vi "Angle Correction PID.vi"(8 "I gain":dbl, 9 "D gain":dbl, 10 "P gain":dbl, 11 "Error In":dbl) -> (3 "Output":dbl)   [LabVIEW 2013, in "ProcessorHelperFunctions.lvlib"]
uses:
  ProcessorHelperFunctions.lvlib
panel:
  out "Error Input":dbl
  out "I accumulated":dbl
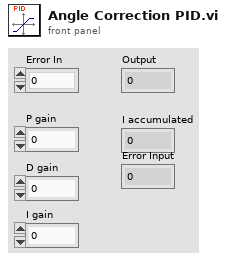
[diagram p1: front panel]
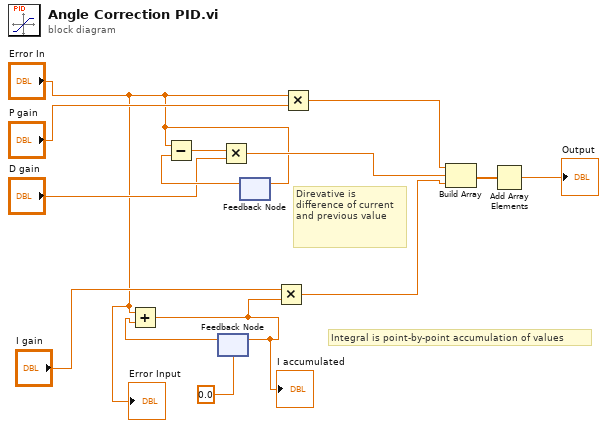
[diagram p0: block diagram]
diagram:
  # "Direvative is difference of current and previous value"
  # "Integral is point-by-point accumulation of values"
  n1 = feedback #1(0.0) -> (w6:dbl)
  n2 = Add(x="Error In", y=w6) -> (x+y=w3:dbl)
  "I accumulated" <- w3
  n3 = feedback-in #1(w3) -> ()
  n4 = feedback-in #2("Error In") -> ()
  n5 = feedback #2() -> (w10:dbl)  [unwired: 1 in]
  n6 = Subtract(x="Error In", y=w10) -> (x-y=w9:dbl)
  n7 = Multiply(x=w9, y="D gain") -> (x*y=w7:dbl)
  n8 = Multiply(x="I gain", y=w3) -> (x*y=w4:dbl)
  n9 = Multiply(x="Error In", y="P gain") -> (x*y=w12:dbl)
  n10 = Build Array(w12, w7, w4) -> (w13:dbl[])
  n11 = Add Array Elements(numeric array=w13) -> (sum=→"Output":dbl)
  "Error Input" <- "Error In"
